vi "ECG AF SPI Input Basic.vi"() -> ()   [LabVIEW 2013]
uses:
  <vilib>/Platform/TimedLoop/XDataNode/timing_clust.ctl
  <vilib>/Platform/TimedLoop/XDataNode/nitl_modes.ctl
  <vilib>/Platform/TimedLoop/XDataNode/wakeup.ctl
  <vilib>/rvi/Emulation/niFpgaSctlEmulationGetInTimedLoop.vi
  <vilib>/rvi/Emulation/niFpgaEmulationReportErrorSimple.vi
  <vilib>/rvi/Emulation/niFpgaGetClockAttributes.vi
  <vilib>/rvi/Emulation/niFpgaCriticalErrorInLSC.vi
  <vilib>/rvi/eio/common/nirviEmuTemplateMethod_errors.vi
  <vilib>/rvi/DataTransferAndStorage/Container/Common/niFpgaContainerGetUniqueNameForEmu.vi
  <vilib>/rvi/DataTransferAndStorage/Container/Common/niFpgaContainerSetEmuInfo.vi
  <vilib>/rvi/eio/common/nirviEmuReportErrorAndStop.vi
  <vilib>/rvi/Analysis/common/codeGenErrors/XNode/niFpgaXNodeCodeGenErrorHandle.vi
  <vilib>/rvi/DataTransferAndStorage/Container/Common/niFpgaContainerExecOnDevCompGetState.vi
  <vilib>/rvi/FIFO/Fifo_Resource/nirvififoEmulationWriteFpgaImpl.vi
  <vilib>/rvi/interface/RandomDataEmulation/nirviRandomDataFPGAFIFO.vi
  <vilib>/rvi/interface/RandomDataEmulation/niFpgaRandomDataHandleErrors.vi
  <vilib>/rvi/FIFO/Fifo_Resource/nirvififoEmulationGetNumberOfElementsToReadFpgaImpl.vi
  <vilib>/rvi/FIFO/Fifo_Resource/nirvififoEmulationReadFpgaImpl.vi
  <vilib>/rvi/Emulation/niFpgaProcessEmulError.vi
  <vilib>/Platform/TimedLoop/XDataNode/XDataNode.xnode
  <vilib>/eio/EIONode/EIONode.xnode
  <vilib>/eio/EIOMethodNode/EIOMethodNode.xnode
  <vilib>/rvi/LocalResourceManager/LocalResourceManager.xnode
  <vilib>/rvi/Analysis/measure/butterworth/XNode/niFpgaButterworthFilter.xnode
  <vilib>/rvi/Analysis/measure/LMRsmpl/XNode/niFPGA Rational Resampler.xnode
  <vilib>/rvi/DataTransferAndStorage/Container/XNode/niFpgaContainer.xnode
  <vilib>/rvi/FIFO/Fifo_Resource/niFpgaFifoEmulationRefIn.vi
  <vilib>/Platform/TimedLoop/XDataNode/XDNodeRunTimeDep.lvlib
  MyFPGACode.lvlib
panel:
  in  "Highpass":bool
  in  "Start 0":bool
  in  "Filter On":bool=TRUE
  in  "Beta":fxp<+/-,32,-12>
  out "Output 8":i16
  out "Output 7":i16
  out "Output 6":i16
  out "Output 5":i16
  out "Output 4":i16
  out "Output 3":i16
  out "Output 2":i16
  out "Output 1":i16
  out "Output 0":i16
  out "Input 8":i16
  out "Input 7":i16
  out "Input 6":i16
  out "Input 5":i16
  out "Input 4":i16
  out "Input 3":i16
  out "Input 2":i16
  out "Input 1":i16
  in  "Local Stop 0":bool
  out "Actual Loop Rate (Ticks)":u32
  out "Late? Latched":bool
  out "Input 0":i16
  in  "Loop Rate (Ticks)":u32=4000
  in  "Reset":bool
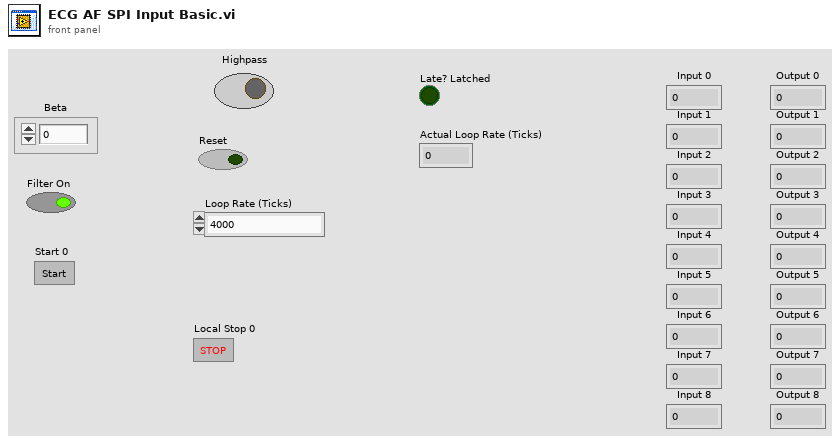
[diagram p1: front panel]
types:
  T1 = typedef "XDNodeRunTimeDep.lvlib/timing_clust.ctl" = cluster{"Expected End [f-1]":u64, "Actual End [f-1]":u64, "Finished Late? [f-1]":bool, "Expected End [i-1]":u64, "Actual End [i-1]":u64, "Finished Late? [i-1]":bool, "Expected Start [i]":u64, "Actual Start [i]":u64, "Expected Start [f]":u64, "Actual Start [f]":u64, "Source Name":string, "Structure Name":string, "Period":i64, "Deadline":i64, "Offset":i64, "Start":i64, "Priority":i32, "Timeout":i32, "Mode":T2, "Wakeup Reason":T3, "Error":errorcluster, "Source Type":string, "Secondary Source Type":string, "Global End Time":u64, "Global Start Time":u64, "Frame Duration":u64, "Iteration Duration":u64, "Assigned CPU":i32, "I/O Scan Engine Mode":u32}
  T2 = typedef "XDNodeRunTimeDep.lvlib/nitl_modes.ctl" = enum32{"No Change", "Process missed periods, maintain original phase", "Discard missed periods, maintain original phase", "Process missed periods, ignore original phase", "Discard missed periods, ignore original phase"}
  T3 = typedef "XDNodeRunTimeDep.lvlib/wakeup.ctl" = enum32{"Normal", "Aborted", "Asynchronous wakeup", "Timing source error", "Timed loop error", "Timeout"}
  T4 = cluster{"X":fxp<+/-,16,16>, "Y":fxp<+/-,16,16>, "Z":fxp<+/-,16,16>}
  T5 = cluster{"[0]":fxp<+/-,16,16>, "[1]":fxp<+/-,16,16>, "[2]":fxp<+/-,16,16>}
  T6 = typedef "MyFPGACode.lvlib/ECG Data Analog.ctl" = cluster{"Channel 0":i16, "Channel 1":i16, "Channel 2":i16, "Channel 3":i16, "Channel 4":i16, "Channel 5":i16, "Channel 6":i16, "Channel 7":i16}
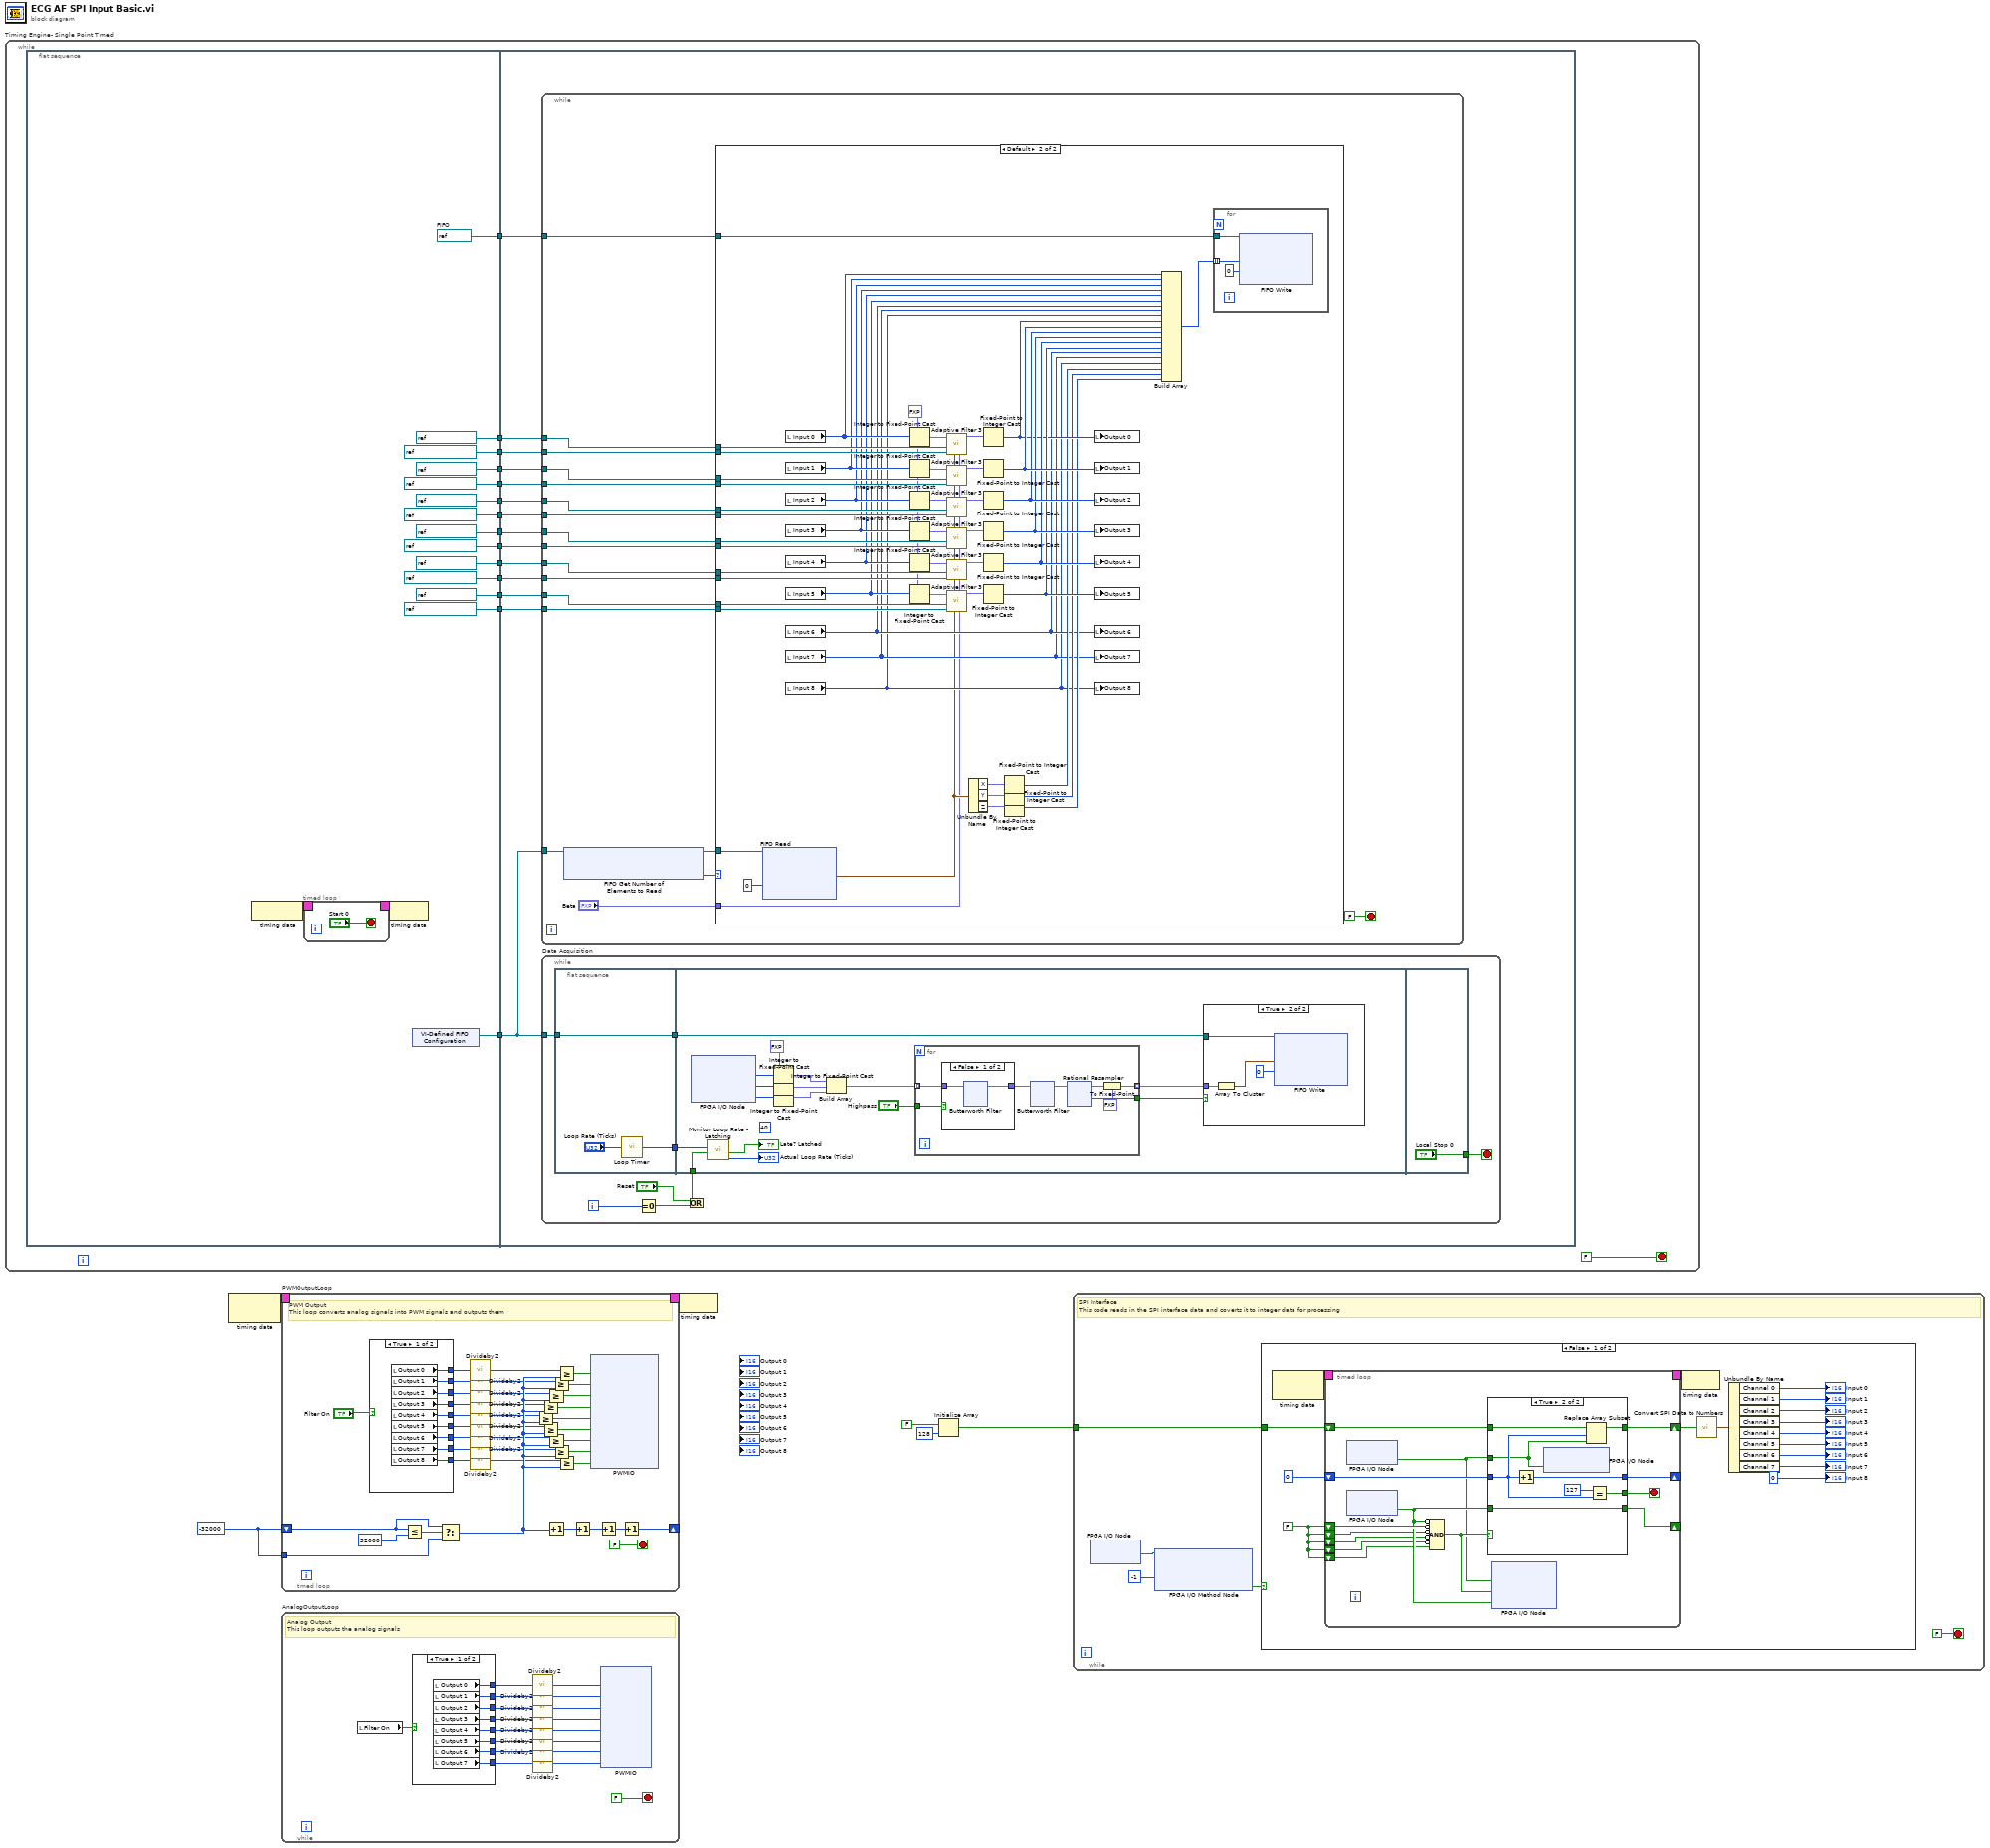
[diagram p0: block diagram]
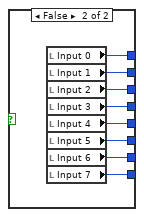
[diagram p2: hidden frame]
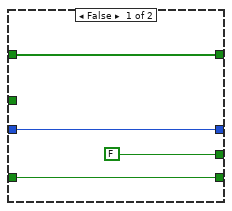
[diagram p3: hidden frame]
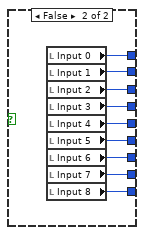
[diagram p5: hidden frame]
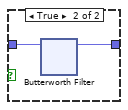
[diagram p7: hidden frame]
diagram:
  w4 = i16 -32000
  n1 = while "Timing Engine- Single Point Timed" {
    stop <- FALSE stop-if-true
    n2 = flat-sequence "MainSeq" {
      tunnel: [w37] -> w20
      tunnel: [refnum<k21> "Filter Taps 0" ("Memory")] -> w19
      tunnel: [refnum<k21> "Filter Weights 1" ("Memory")] -> w18
      tunnel: [refnum<k21> "Filter Taps 1" ("Memory")] -> w17
      tunnel: [refnum<k21> "Filter Weights 2" ("Memory")] -> w16
      tunnel: [refnum<k21> "Filter Taps 2" ("Memory")] -> w15
      tunnel: [refnum<k21> "Filter Taps 3" ("Memory")] -> w14
      tunnel: [refnum<k21> "Filter Weights 3" ("Memory")] -> w13
      tunnel: [refnum<k21> "Filter Weights 4" ("Memory")] -> w12
      tunnel: [refnum<k21> "Filter Taps 4" ("Memory")] -> w11
      tunnel: [refnum<k21> "Filter Weights 5" ("Memory")] -> w10
      tunnel: [refnum<k21> "Filter Taps 5" ("Memory")] -> w9
      tunnel: [refnum<k21> "Filter Weights 0" ("Memory")] -> w8
      tunnel: [w22] -> w7
      tunnel: w20 -> [w56]
      tunnel: w19 -> [w55]
      tunnel: w18 -> [w53]
      tunnel: w17 -> [w52]
      tunnel: w16 -> [w51]
      tunnel: w15 -> [w50]
      tunnel: w14 -> [w49]
      tunnel: w13 -> [w48]
      tunnel: w12 -> [w47]
      tunnel: w11 -> [w46]
      tunnel: w10 -> [w45]
      tunnel: w9 -> [w44]
      tunnel: w8 -> [w54]
      tunnel: w7 -> [w43]
      frame #0 {
        w22 = refnum<k21> "FIFO"  # FIFO
        n3 = node-c288 ("Input Node")() -> (w36:T1)
        n4 = timed-loop "initWait" {
          timing: w36 -> [_]
          timing-out: [_] -> w35
          stop <- "Start 0" stop-if-true
        }
        n5 = node-c288 ("Output Node")(w35) -> ()
        n6 = xnode "VI-Defined FIFO Configuration"() -> ("FIFO Out"=w37:refnum<k21>)
      }
      frame #1 {
        n7 = while {
          tunnel: w56 -> [w74]
          tunnel: w55 -> [w70]
          tunnel: w54 -> [w69]
          tunnel: w53 -> [w68]
          tunnel: w52 -> [w67]
          tunnel: w51 -> [w66]
          tunnel: w50 -> [w65]
          tunnel: w49 -> [w64]
          tunnel: w48 -> [w63]
          tunnel: w47 -> [w62]
          tunnel: w46 -> [w61]
          tunnel: w45 -> [w60]
          tunnel: w44 -> [w59]
          tunnel: w43 -> [w57]
          stop <- FALSE stop-if-true
          n8 = xnode ("FIFO Get Number of Elements to Read")("FIFO In"=w74) -> ("Number of Elements to Read"=w73:u32, "FIFO Out"=w72:refnum<k21>)
          n9 = case shown="Default" w73 {
            tunnel: w72 -> [_ w126]
            tunnel: "Beta" -> [_ w90]
            tunnel: w70 -> [_ w124]
            tunnel: w69 -> [_ w113]
            tunnel: w68 -> [_ w114]
            tunnel: w67 -> [_ w123]
            tunnel: w66 -> [_ w122]
            tunnel: w65 -> [_ w121]
            tunnel: w64 -> [_ w120]
            tunnel: w63 -> [_ w119]
            tunnel: w62 -> [_ w118]
            tunnel: w61 -> [_ w117]
            tunnel: w60 -> [_ w116]
            tunnel: w59 -> [_ w115]
            tunnel: w57 -> [_ w100]
            frame 0 {
            }
            frame Default {
              w112 = fxp<+/-,16,16> 0.0 ("fixed-point type")
              n10 = xnode ("FIFO Read")("Timeout"=0, "FIFO In"=w126) -> ("Element"=w91:T4)  [unwired: 2 out]
              n11 = local read "Input 0"() -> (w111:i16)
              n12 = local read "Input 1"() -> (w110:i16)
              n13 = local read "Input 2"() -> (w109:i16)
              n14 = local read "Input 3"() -> (w108:i16)
              n15 = local read "Input 4"() -> (w107:i16)
              n16 = local read "Input 5"() -> (w106:i16)
              n17 = local read "Input 6"() -> (w94:i16)
              n18 = local read "Input 7"() -> (w93:i16)
              n19 = local read "Input 8"() -> (w92:i16)
              n20 = Integer to Fixed-Point Cast(fixed-point type=w112, integer=w111) -> (fixed-point=w89:fxp<+/-,16,16>)
              n21 = Integer to Fixed-Point Cast(fixed-point type=w112, integer=w110) -> (fixed-point=w88:fxp<+/-,16,16>)
              n22 = Integer to Fixed-Point Cast(fixed-point type=w112, integer=w109) -> (fixed-point=w78:fxp<+/-,16,16>)
              n23 = Integer to Fixed-Point Cast(fixed-point type=w112, integer=w108) -> (fixed-point=w87:fxp<+/-,16,16>)
              n24 = Integer to Fixed-Point Cast(fixed-point type=w112, integer=w107) -> (fixed-point=w86:fxp<+/-,16,16>)
              n25 = Integer to Fixed-Point Cast(fixed-point type=w112, integer=w106) -> (fixed-point=w85:fxp<+/-,16,16>)
              n26 = call "Adaptive Filter 3.vi"("Beta"=w90, "Noise"=w91, "Weights"=w113, "Taps"=w124, "Input"=w89) -> ("Error Out"=w84:fxp<+/-,16,16>)  [unwired: 6 in]
              n27 = call "Adaptive Filter 3.vi"("Beta"=w90, "Noise"=w91, "Weights"=w114, "Taps"=w123, "Input"=w88) -> ("Error Out"=w83:fxp<+/-,16,16>)  [unwired: 6 in]
              n28 = call "Adaptive Filter 3.vi"("Beta"=w90, "Noise"=w91, "Weights"=w122, "Taps"=w121, "Input"=w78) -> ("Error Out"=w82:fxp<+/-,16,16>)  [unwired: 6 in]
              n29 = call "Adaptive Filter 3.vi"("Beta"=w90, "Noise"=w91, "Weights"=w119, "Taps"=w120, "Input"=w87) -> ("Error Out"=w81:fxp<+/-,16,16>)  [unwired: 6 in]
              n30 = call "Adaptive Filter 3.vi"("Beta"=w90, "Noise"=w91, "Weights"=w118, "Taps"=w117, "Input"=w86) -> ("Error Out"=w80:fxp<+/-,16,16>)  [unwired: 6 in]
              n31 = call "Adaptive Filter 3.vi"("Beta"=w90, "Noise"=w91, "Weights"=w116, "Taps"=w115, "Input"=w85) -> ("Error Out"=w79:fxp<+/-,16,16>)  [unwired: 6 in]
              n32 = Unbundle By Name(w91) -> ("X"=w77:fxp<+/-,16,16>, "Y"=w76:fxp<+/-,16,16>, "Z"=w75:fxp<+/-,16,16>)
              n33 = Fixed-Point to Integer Cast(1:w84) -> (0:w98:i16)
              n34 = Fixed-Point to Integer Cast(1:w83) -> (0:w105:i16)
              n35 = Fixed-Point to Integer Cast(1:w82) -> (0:w104:i16)
              n36 = Fixed-Point to Integer Cast(1:w81) -> (0:w103:i16)
              n37 = Fixed-Point to Integer Cast(1:w80) -> (0:w102:i16)
              n38 = Fixed-Point to Integer Cast(1:w79) -> (0:w101:i16)
              n39 = Fixed-Point to Integer Cast(1:w77) -> (0:w97:i16)
              n40 = Fixed-Point to Integer Cast(1:w76) -> (0:w96:i16)
              n41 = Fixed-Point to Integer Cast(1:w75) -> (0:w95:i16)
              n42 = local write "Output 0"(w98) -> ()
              n43 = local write "Output 1"(w105) -> ()
              n44 = local write "Output 2"(w104) -> ()
              n45 = local write "Output 3"(w103) -> ()
              n46 = local write "Output 4"(w102) -> ()
              n47 = local write "Output 5"(w101) -> ()
              n48 = local write "Output 6"(w94) -> ()
              n49 = local write "Output 7"(w93) -> ()
              n50 = local write "Output 8"(w92) -> ()
              n51 = Build Array(w111, w110, w109, w108, w107, w106, w94, w93, w92, w98, w105, w104, w103, w102, w101, w94, w93, w92, w97, w96, w95) -> (w99:i16[])
              n52 = for {
                tunnel: w100 -> [w129]
                tunnel: w99 -> [w128] mode=indexing
                n53 = xnode ("FIFO Write")("Element"=w128, "Timeout"=0, "FIFO In"=w129) -> ()  [unwired: 2 out]
              }
            }
          }
        }
        n54 = while "Data Acquisition" {
          tunnel: w56 -> [w132]
          i -> [w130]
          stop <- w137 stop-if-true
          n55 = flat-sequence "Data Acquisition Sequence" {
            tunnel: ["Loop Rate (Ticks)"] -> w136
            tunnel: w132 -> [w139]
            tunnel: [w139] -> w131
            tunnel: w136 -> [w153]
            tunnel: w133 -> [w154]
            tunnel: w131 -> [w151]
            tunnel: ["Local Stop 0"] -> w137
            frame #0 {
              n56 = call "Loop Timer"("Count(Ticks)"="Loop Rate (Ticks)") -> ()  [unwired: 1 out]
            }
            frame #1 {
              (unwired) i16 40 ("y")
              w149 = fxp<+/-,16,16> 0.0 ("fixed-point type")
              n57 = xnode "FPGA I/O Node"() -> ("X Gradient"=w143:i16, "Y Gradient"=w142:i16, "Z Gradient"=w141:i16)  [unwired: 3 in, 3 out]
              n58 = call "Monitor Loop Rate - Latching.vi"("Reset"=w154, "Count(Ticks)"=w153) -> ("Actual Loop Rate (Ticks)"=→"Actual Loop Rate (Ticks)":u32, "Late? (Latched)"=→"Late? Latched":bool)  [unwired: 7 in, 1 out]
              n59 = Integer to Fixed-Point Cast(fixed-point type=w149, integer=w143) -> (fixed-point=w145:fxp<+/-,16,16>)
              n60 = Integer to Fixed-Point Cast(fixed-point type=w149, integer=w142) -> (fixed-point=w146:fxp<+/-,16,16>)
              n61 = Integer to Fixed-Point Cast(fixed-point type=w149, integer=w141) -> (fixed-point=w144:fxp<+/-,16,16>)
              n62 = Build Array(w145, w146, w144) -> (w147:fxp<+/-,16,16>[])
              n63 = for {
                tunnel: w147 -> [w161] mode=indexing
                tunnel: [w158] -> w152 mode=indexing
                tunnel: [w159] -> w150
                tunnel: "Highpass" -> [w156]
                n64 = case shown="False" w156 {
                  tunnel: [w164 w176] -> w163
                  tunnel: w161 -> [w165 w175]
                  frame False {
                    n65 = xnode "Butterworth Filter"("input data"=w165) -> ("output data"=w164:fxp<+/-,16,16>)  [unwired: 2 in, 1 out]
                  }
                  frame True {
                    n66 = xnode "Butterworth Filter"("input data"=w175) -> ("output data"=w176:fxp<+/-,16,16>)  [unwired: 2 in, 1 out]
                  }
                }
                n67 = xnode "Butterworth Filter"("input data"=w163) -> ("output data"=w162:fxp<+/-,16,16>)  [unwired: 2 in, 1 out]
                n68 = xnode "Rational Resampler"("input data"=w162) -> ("output data"=w160:fxp<+/-,18,16>, "output valid"=w159:bool)  [unwired: 1 out]
                n69 = To Fixed-Point(fixed-point type=fxp<+/-,16,16> 0.0, number=w160) -> (fixed-point=w158:fxp<+/-,16,16>)
              }
              n70 = case shown="True" w150 {
                tunnel: w152 -> [_ w248]
                tunnel: w151 -> [_ w247]
                frame False {
                }
                frame True {
                  n71 = Array To Cluster(array=w248) -> (cluster=w246:T5)
                  n72 = xnode ("FIFO Write")("Element"=w246, "Timeout"=0, "FIFO In"=w247) -> ()  [unwired: 2 out]
                }
              }
            }
            frame #2 {
            }
          }
          n73 = Equal To 0?(x=w130) -> (x = 0?=w135:bool)
          n74 = Or(x="Reset", y=w135) -> (x .or. y?=w133:bool)
        }
      }
    }
  }
  n75 = node-c288 ("Input Node")() -> (w6:T1)  [unwired: 1 in]
  n76 = timed-loop "PWMOutputLoop" {
    timing: w6 -> [_]
    timing-out: [_] -> w5
    shift-right: [w266] -> _
    shift-left: w4 -> [w284]
    tunnel: w4 -> [w271]
    stop <- FALSE stop-if-true
    # "PWM Output\nThis loop converts analog signals into PWM signals and outputs them"
    n77 = case shown="True" "Filter On" {
      tunnel: [w296 w305] -> w269
      tunnel: [w295 w304] -> w268
      tunnel: [w294 w303] -> w262
      tunnel: [w293 w302] -> w263
      tunnel: [w292 w301] -> w259
      tunnel: [w291 w300] -> w258
      tunnel: [w290 w299] -> w260
      tunnel: [w289 w298] -> w261
      tunnel: [w288 w297] -> w257
      frame True {
        n78 = local read "Output 0"() -> (w296:i16)
        n79 = local read "Output 1"() -> (w295:i16)
        n80 = local read "Output 2"() -> (w293:i16)
        n81 = local read "Output 3"() -> (w294:i16)
        n82 = local read "Output 4"() -> (w289:i16)
        n83 = local read "Output 5"() -> (w290:i16)
        n84 = local read "Output 6"() -> (w292:i16)
        n85 = local read "Output 7"() -> (w291:i16)
        n86 = local read "Output 8"() -> (w288:i16)
      }
      frame False {
        n87 = local read "Input 0"() -> (w305:i16)
        n88 = local read "Input 1"() -> (w304:i16)
        n89 = local read "Input 2"() -> (w302:i16)
        n90 = local read "Input 3"() -> (w303:i16)
        n91 = local read "Input 4"() -> (w298:i16)
        n92 = local read "Input 5"() -> (w299:i16)
        n93 = local read "Input 6"() -> (w301:i16)
        n94 = local read "Input 7"() -> (w300:i16)
        n95 = local read "Input 8"() -> (w297:i16)
      }
    }
    n96 = Less Or Equal?(x=w284, y=i16 32000 ("Period")) -> (x <= y?=w285:bool)
    n97 = Select(t=w284, s=w285, f=w271) -> (s? t:f=w274:i16)
    n98 = call "Divideby2.vi"("Input"=w269) -> ("Output"=w265:i16)
    n99 = call "Divideby2.vi"("Input"=w268) -> ("Output"=w264:i16)
    n100 = call "Divideby2.vi"("Input"=w263) -> ("Output"=w250:i16)
    n101 = call "Divideby2.vi"("Input"=w262) -> ("Output"=w251:i16)
    n102 = call "Divideby2.vi"("Input"=w261) -> ("Output"=w252:i16)
    n103 = call "Divideby2.vi"("Input"=w260) -> ("Output"=w253:i16)
    n104 = call "Divideby2.vi"("Input"=w259) -> ("Output"=w254:i16)
    n105 = call "Divideby2.vi"("Input"=w258) -> ("Output"=w255:i16)
    n106 = call "Divideby2.vi"("Input"=w257) -> ("Output"=w256:i16)
    n107 = Greater Or Equal?(x=w252, y=w274) -> (x >= y?=w278:bool)
    n108 = Greater Or Equal?(x=w251, y=w274) -> (x >= y?=w279:bool)
    n109 = Greater Or Equal?(x=w253, y=w274) -> (x >= y?=w277:bool)
    n110 = Greater Or Equal?(x=w250, y=w274) -> (x >= y?=w280:bool)
    n111 = Greater Or Equal?(x=w254, y=w274) -> (x >= y?=w276:bool)
    n112 = Increment(x=w274) -> (x+1=w283:i16)
    n113 = Greater Or Equal?(x=w264, y=w274) -> (x >= y?=w281:bool)
    n114 = Greater Or Equal?(x=w255, y=w274) -> (x >= y?=w275:bool)
    n115 = Greater Or Equal?(x=w265, y=w274) -> (x >= y?=w282:bool)
    n116 = Greater Or Equal?(x=w256, y=w274) -> (x >= y?=w273:bool)
    n117 = Increment(x=w283) -> (x+1=w270:i16)
    n118 = xnode ("PWMIO")("ECG0 PWM"=w282, "ECG1 PWM"=w281, "ECG2 PWM"=w280, "ECG3 PWM"=w279, "ECG4 PWM"=w278, "ECG5 PWM"=w277, "ECG6 PWM"=w276, "ECG7 PWM"=w275, "ECG8 PWM"=w273) -> ()  [unwired: 9 in, 9 out]
    n119 = Increment(x=w270) -> (x+1=w267:i16)
    n120 = Increment(x=w267) -> (x+1=w266:i16)
  }
  n121 = while "AnalogOutputLoop" {
    stop <- FALSE stop-if-true
    # "Analog Output\nThis loop outputs the analog signals"
    n122 = local read "Filter On"() -> (w324:bool)
    n123 = case shown="True" w324 {
      tunnel: [w333 w341] -> w323
      tunnel: [w332 w340] -> w322
      tunnel: [w331 w339] -> w320
      tunnel: [w330 w338] -> w321
      tunnel: [w329 w337] -> w317
      tunnel: [w328 w336] -> w316
      tunnel: [w327 w335] -> w318
      tunnel: [w326 w334] -> w319
      frame True {
        n124 = local read "Output 0"() -> (w333:i16)
        n125 = local read "Output 1"() -> (w332:i16)
        n126 = local read "Output 2"() -> (w330:i16)
        n127 = local read "Output 3"() -> (w331:i16)
        n128 = local read "Output 4"() -> (w326:i16)
        n129 = local read "Output 5"() -> (w327:i16)
        n130 = local read "Output 6"() -> (w329:i16)
        n131 = local read "Output 7"() -> (w328:i16)
      }
      frame False {
        n132 = local read "Input 0"() -> (w341:i16)
        n133 = local read "Input 1"() -> (w340:i16)
        n134 = local read "Input 2"() -> (w338:i16)
        n135 = local read "Input 3"() -> (w339:i16)
        n136 = local read "Input 4"() -> (w334:i16)
        n137 = local read "Input 5"() -> (w335:i16)
        n138 = local read "Input 6"() -> (w337:i16)
        n139 = local read "Input 7"() -> (w336:i16)
      }
    }
    n140 = call "Divideby2.vi"("Input"=w323) -> ("Output"=w315:i16)
    n141 = call "Divideby2.vi"("Input"=w322) -> ("Output"=w314:i16)
    n142 = call "Divideby2.vi"("Input"=w321) -> ("Output"=w313:i16)
    n143 = call "Divideby2.vi"("Input"=w320) -> ("Output"=w312:i16)
    n144 = call "Divideby2.vi"("Input"=w319) -> ("Output"=w311:i16)
    n145 = call "Divideby2.vi"("Input"=w318) -> ("Output"=w310:i16)
    n146 = call "Divideby2.vi"("Input"=w317) -> ("Output"=w309:i16)
    n147 = call "Divideby2.vi"("Input"=w316) -> ("Output"=w308:i16)
    n148 = xnode ("PWMIO")("ECG0"=w315, "ECG1"=w314, "ECG2"=w313, "ECG3"=w312, "ECG4"=w311, "ECG5"=w310, "ECG6"=w309, "ECG7"=w308) -> ()  [unwired: 8 in, 8 out]
  }
  n149 = node-c288 ("Output Node")(w5) -> ()
  n150 = Initialize Array(FALSE, 128 ("dimension size")) -> (w3:bool[])
  n151 = while {
    tunnel: w3 -> [w342]
    stop <- FALSE stop-if-true
    # "SPI Interface\nThis code reads in the SPI interface data and coverts it to integer data for processing"
    n152 = xnode "FPGA I/O Node"() -> ("FPGA I/O Out"=w343:refnum<k21>)  [unwired: 1 in, 1 out]
    n153 = xnode "FPGA I/O Method Node"("FPGA I/O In"=w343, "Timeout"=-1) -> ("Timed Out"=w345:bool)  [unwired: 1 out]
    n154 = case shown="False" w345 {
      tunnel: w342 -> [w362 _]
      frame False {
        w358 = FALSE
        n155 = node-c288() -> (w361:T1)  [unwired: 1 in]
        n156 = timed-loop {
          shift-right: [w374] -> w357
          shift-left: w362 -> [w375]
          timing: w361 -> [_]
          timing-out: [_] -> w360
          shift-right: [w370] -> _
          shift-left: w358 -> [w373]
          shift-right: [w371] -> _
          shift-left: u8 0 -> [w372]
          shift-left: w358 -> [w366]
          shift-left: w358 -> [w365]
          shift-left: w358 -> [w364]
          shift-left: w358 -> [w363]
          stop <- w376 stop-if-true
          n157 = xnode "FPGA I/O Node"() -> ("MOSI"=w367:bool)  [unwired: 1 in, 1 out]
          n158 = xnode "FPGA I/O Node"() -> ("SCLK"=w369:bool)  [unwired: 1 in, 1 out]
          n159 = Compound Arithmetic op=AND(invert w369, invert w373, invert w366, invert w365, invert w364, w363) -> (w368:bool)
          n160 = case shown="True" w368 {
            tunnel: [FALSE w387] -> w376
            tunnel: w375 -> [w377 w386]
            tunnel: [w377 w385] -> w374
            tunnel: w372 -> [w380 w384]
            tunnel: [w380 w383] -> w371
            tunnel: w369 -> [w379 w382]
            tunnel: [w379 w382] -> w370
            tunnel: w367 -> [_ w381]
            frame False {
            }
            frame True {
              n161 = Increment(x=w384) -> (x+1=w383:u8)
              n162 = xnode "FPGA I/O Node"("MOSI Data"=w381) -> ()  [unwired: 1 in, 1 out]
              n163 = Replace Array Subset(array=w386, new element=w381, index=w384) -> (w385:bool[])
              n164 = Equal?(x=u8 127, y=w384) -> (x = y?=w387:bool)
            }
          }
          n165 = xnode "FPGA I/O Node"("MOSI Out"=w367, "SCLK Edge"=w368, "SCLK Out"=w369) -> ()  [unwired: 3 in, 3 out]
        }
        n166 = node-c288(w360) -> ()
        n167 = call "Convert SPI Data to Numbers.vi"("Data In"=w357) -> ("ECG Data"=w356:T6)
        n168 = Unbundle By Name(w356) -> ("Channel 0"=→"Input 0":i16, "Channel 1"=→"Input 1":i16, "Channel 2"=→"Input 2":i16, "Channel 3"=→"Input 3":i16, "Channel 4"=→"Input 4":i16, "Channel 5"=→"Input 5":i16, "Channel 6"=→"Input 6":i16, "Channel 7"=→"Input 7":i16)
        "Input 8" <- i16 0 ("Input 8")
      }
      frame True {
      }
    }
  }
